vi "LM Numeric Gradient.vi"(6 "order":i32(ring)=1 items=["ORDER 1"=1, "ORDER 2"=2, "ORDER 4"=4], 7 "model function":T1, 8 "error in (no error)":errorcluster, 9 "X":dbl[](array[numeric]), 10 "f(X)":dbl[](array[numeric]), 11 "a":dbl[](array[numeric])) -> (0 "error out":errorcluster, 2 "number of function evaluations":i32, 3 "gradient":dbl[][](array[numeric]))   [LabVIEW 2010, in "NI_Gmath.lvlib"]
uses:
  NI_Gmath.lvlib
  LM model function.ctl
  LM model function reference.ctl
  LM_output select.ctl
  fpuIEEE64_finiteDiffConstants.ctl
panel:
  in  "stepsize (h)":dbl
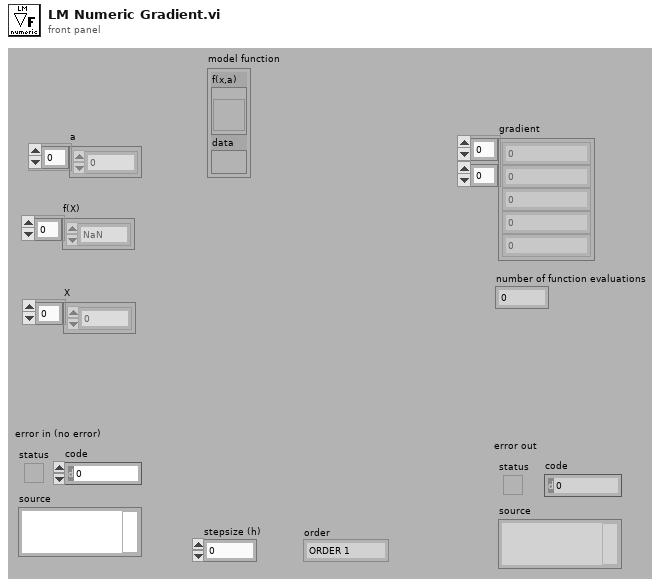
[diagram p1: front panel]
types:
  T1 = typedef "NI_Gmath.lvlib/LM model function.ctl" = cluster{"f(x,a)":T2, "data":variant}
  T2 = typedef "NI_Gmath.lvlib/LM model function reference.ctl" = refnum<vi>
  T3 = typedef "NI_Gmath.lvlib/LM_output select.ctl" = cluster{"model function":bool, "gradient":bool}
  T4 = typedef "NI_Gmath.lvlib/fpuIEEE64_finiteDiffConstants.ctl" = dbl
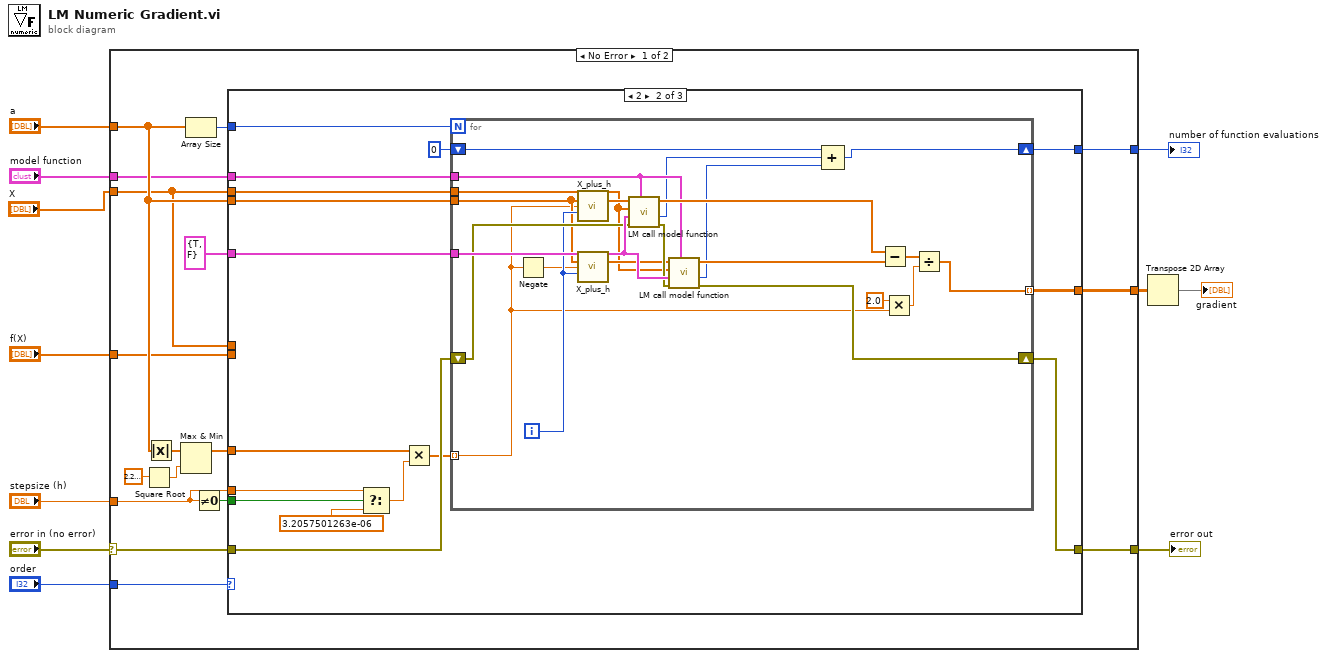
[diagram p0: block diagram]
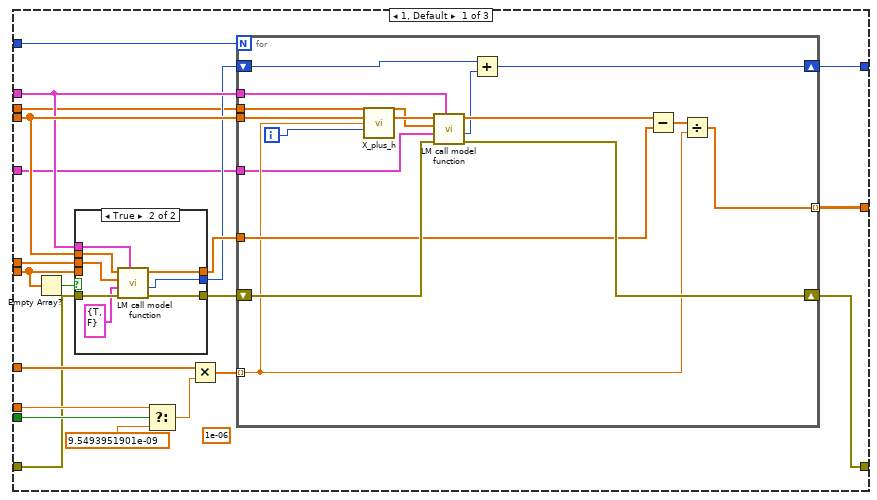
[diagram p2: hidden frame]
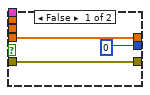
[diagram p3: hidden frame]
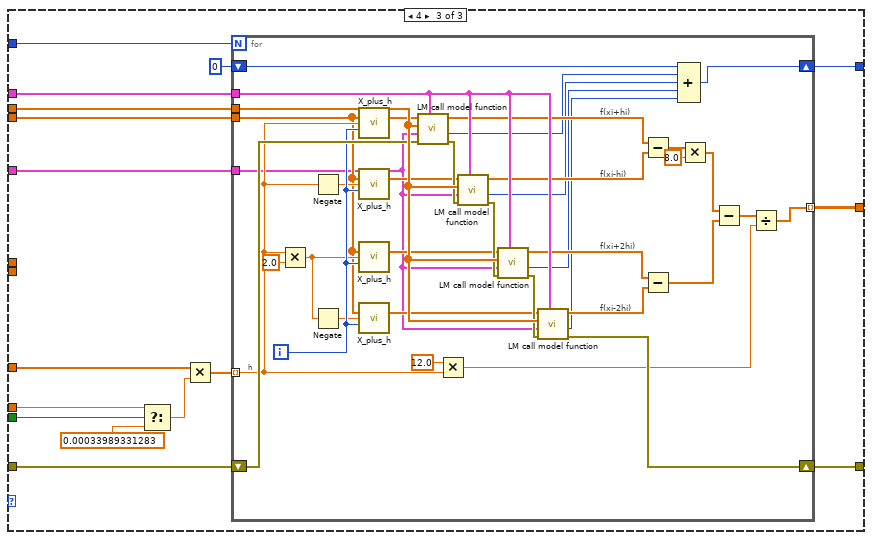
[diagram p4: hidden frame]
diagram:
  n1 = case shown="No Error" "error in (no error)" {
    selector: "error in (no error)" -> [w20 w168]
    tunnel: "a" -> [w28 _]
    tunnel: [w27 _] -> w10
    tunnel: "order" -> [w26 _]
    tunnel: "f(X)" -> [w24 _]
    tunnel: "stepsize (h)" -> [w23 _]
    tunnel: [w21 w168] -> w6
    tunnel: "model function" -> [w19 _]
    tunnel: [w18 _] -> w3
    tunnel: "X" -> [w17 _]
    frame No Error {
      n2 = Square Root(x=2.220446049250313e-16) -> (sqrt(x)=w14:dbl)
      n3 = Absolute Value(x=w28) -> (abs(x)=w13:dbl[])
      n4 = Max & Min(x=w13, y=w14) -> (max(x,y)=w12:dbl[])  [unwired: 1 out]
      n5 = Array Size(array=w28) -> (size(s)=w25:i32)
      n6 = Not Equal To 0?(x=w23) -> (x != 0?=w22:bool)
      n7 = case shown="2" w26 {
        tunnel: w28 -> [w45 w91 w130]
        tunnel: w20 -> [w38 w92 w121]
        tunnel: [w48 w90 w129] -> w27
        tunnel: w25 -> [w47 w89 w128]
        tunnel: w24 -> [w31 _ _]
        tunnel: w23 -> [w44 w86 w126]
        tunnel: w22 -> [w43 w87 w125]
        tunnel: w12 -> [w40 w85 w123]
        tunnel: [w49 w82 w120] -> w21
        tunnel: w19 -> [w37 w81 w119]
        tunnel: [w36 w79 w118] -> w18
        tunnel: w17 -> [w34 _ _]
        tunnel: w17 -> [w33 w78 w116]
        tunnel: T3 {"model function"=TRUE, "gradient"=FALSE} ("output control") -> [w30 w77 w115]
        frame 1, Default {
          (unwired) 1e-06
          w42 = T4 9.5493951901e-09 items=["H_FINITE_DIFF_1"=9.5493951901e-09, "H_FINITE_DIFF_2"=3.2057501263e-06, "H_FINITE_DIFF_4"=0.00033989331283, "H_FINITE_DIFF_K_1"=2.8120287999e-06, "H_FINITE_DIFF_K_2"=9.1341513557e-05, "H_FINITE_DIFF_K_3"=0.00045180790895, "H_FINITE_DIFF_K_4"=0.0014917421406] ("fpuIEEE64")
          n8 = Empty Array?(array=w31) -> (empty?=w32:bool)
          n9 = case shown="True" w32 {
            tunnel: [w52 w58] -> w46
            tunnel: w45 -> [_ w56]
            tunnel: w31 -> [w52 _]
            tunnel: w38 -> [w51 w60]
            tunnel: [w51 w59] -> w39
            tunnel: w37 -> [_ w57]
            tunnel: [0 ("number of function evaluations") w54] -> w35
            tunnel: w34 -> [_ w55]
            frame False {
            }
            frame True {
              n10 = call "LM call model function.vi"("model function"=w57, "error in (no error)"=w60, "output control"=T3 {"model function"=TRUE, "gradient"=FALSE}, "X"=w55, "a"=w56) -> ("error out"=w59:errorcluster, "number of function evaluations"=w54:i32, "f(X)"=w58:dbl[])  [unwired: 3 in, 1 out]
            }
          }
          n11 = Select(t=w44, s=w43, f=w42) -> (s? t:f=w41:T4)
          n12 = Multiply(x=w40, y=w41) -> (x*y=w29:T4[])
          n13 = for {
            N: w47 -> [_]
            tunnel: w45 -> [w70]
            tunnel: [w74] -> w48 mode=indexing
            tunnel: w46 -> [w72]
            tunnel: w29 -> [w69] mode=indexing
            shift-right: [w75] -> w49
            shift-left: w39 -> [w76]
            tunnel: w37 -> [w66]
            shift-right: [w64] -> w36
            shift-left: w35 -> [w65]
            tunnel: w33 -> [w63]
            tunnel: w30 -> [w61]
            i -> [w71]
            n14 = call "X_plus_h.vi"("X"=w70, "h"=w69, "i"=w71) -> ("Xi+h"=w68:dbl[])  [unwired: 12 in]
            n15 = call "LM call model function.vi"("model function"=w66, "error in (no error)"=w76, "output control"=w61, "X"=w63, "a"=w68) -> ("error out"=w75:errorcluster, "number of function evaluations"=w62:i32, "f(X)"=w67:dbl[])  [unwired: 3 in, 1 out]
            n16 = Add(x=w65, y=w62) -> (x+y=w64:i32)
            n17 = Subtract(x=w67, y=w72) -> (x-y=w73:dbl[])
            n18 = Divide(x=w73, y=w69) -> (x/y=w74:T4[])
          }
        }
        frame 2 {
          w88 = T4 3.2057501263e-06 items=["H_FINITE_DIFF_1"=9.5493951901e-09, "H_FINITE_DIFF_2"=3.2057501263e-06, "H_FINITE_DIFF_4"=0.00033989331283, "H_FINITE_DIFF_K_1"=2.8120287999e-06, "H_FINITE_DIFF_K_2"=9.1341513557e-05, "H_FINITE_DIFF_K_3"=0.00045180790895, "H_FINITE_DIFF_K_4"=0.0014917421406] ("fpuIEEE64")
          n19 = Select(t=w86, s=w87, f=w88) -> (s? t:f=w84:T4)
          n20 = Multiply(x=w85, y=w84) -> (x*y=w83:T4[])
          n21 = for {
            N: w89 -> [_]
            tunnel: w91 -> [w105]
            tunnel: [w107] -> w90 mode=indexing
            tunnel: w83 -> [w104] mode=indexing
            shift-right: [w112] -> w82
            shift-left: w92 -> [w111]
            tunnel: w81 -> [w100]
            shift-right: [w98] -> w79
            shift-left: 0 -> [w99]
            tunnel: w78 -> [w95]
            tunnel: w77 -> [w114]
            i -> [w110]
            n22 = Negate(x=w104) -> (-x=w103:T4)
            n23 = call "X_plus_h.vi"("X"=w105, "h"=w104, "i"=w110) -> ("Xi+h"=w96:dbl[])  [unwired: 12 in]
            n24 = call "X_plus_h.vi"("X"=w105, "h"=w103, "i"=w110) -> ("Xi+h"=w97:dbl[])  [unwired: 12 in]
            n25 = call "LM call model function.vi"("model function"=w100, "error in (no error)"=w111, "output control"=w114, "X"=w95, "a"=w96) -> ("error out"=w113:errorcluster, "number of function evaluations"=w94:i32, "f(X)"=w102:dbl[])  [unwired: 3 in, 1 out]
            n26 = call "LM call model function.vi"("model function"=w100, "error in (no error)"=w113, "output control"=w114, "X"=w95, "a"=w97) -> ("error out"=w112:errorcluster, "number of function evaluations"=w93:i32, "f(X)"=w101:dbl[])  [unwired: 3 in, 1 out]
            n27 = Compound Arithmetic op=ADD(w99, w94, w93) -> (w98:i32)
            n28 = Subtract(x=w102, y=w101) -> (x-y=w106:dbl[])
            n29 = Multiply(x=2.0, y=w104) -> (x*y=w108:T4)
            n30 = Divide(x=w106, y=w108) -> (x/y=w107:T4[])
          }
        }
        frame 4 {
          w127 = T4 0.00033989331283 items=["H_FINITE_DIFF_1"=9.5493951901e-09, "H_FINITE_DIFF_2"=3.2057501263e-06, "H_FINITE_DIFF_4"=0.00033989331283, "H_FINITE_DIFF_K_1"=2.8120287999e-06, "H_FINITE_DIFF_K_2"=9.1341513557e-05, "H_FINITE_DIFF_K_3"=0.00045180790895, "H_FINITE_DIFF_K_4"=0.0014917421406] ("fpuIEEE64")
          n31 = Select(t=w126, s=w125, f=w127) -> (s? t:f=w124:T4)
          n32 = Multiply(x=w123, y=w124) -> (x*y=w122:T4[])
          n33 = for {
            N: w128 -> [_]
            tunnel: w130 -> [w146]
            tunnel: [w152] -> w129 mode=indexing
            tunnel: w122 -> [w149] mode=indexing
            shift-right: [w164] -> w120
            shift-left: w121 -> [w165]
            tunnel: w119 -> [w166]
            shift-right: [w140] -> w118
            shift-left: 0 -> [w141]
            tunnel: w116 -> [w167]
            tunnel: w115 -> [w131]
            i -> [w160]
            # "h"
            # "f(xi-2hi)"
            # "f(xi+2hi)"
            # "f(xi-hi)"
            # "f(xi+hi)"
            n34 = Multiply(x=w149, y=2.0) -> (x*y=w147:T4)
            n35 = Negate(x=w149) -> (-x=w151:T4)
            n36 = Negate(x=w147) -> (-x=w148:T4)
            n37 = call "X_plus_h.vi"("X"=w146, "h"=w149, "i"=w160) -> ("Xi+h"=w139:dbl[])  [unwired: 12 in]
            n38 = call "X_plus_h.vi"("X"=w146, "h"=w151, "i"=w160) -> ("Xi+h"=w138:dbl[])  [unwired: 12 in]
            n39 = call "X_plus_h.vi"("X"=w146, "h"=w147, "i"=w160) -> ("Xi+h"=w137:dbl[])  [unwired: 12 in]
            n40 = call "X_plus_h.vi"("X"=w146, "h"=w148, "i"=w160) -> ("Xi+h"=w136:dbl[])  [unwired: 12 in]
            n41 = call "LM call model function.vi"("model function"=w166, "error in (no error)"=w165, "output control"=w131, "X"=w167, "a"=w139) -> ("error out"=w161:errorcluster, "number of function evaluations"=w135:i32, "f(X)"=w145:dbl[])  [unwired: 3 in, 1 out]
            n42 = Multiply(x=12.0, y=w149) -> (x*y=w154:T4)
            n43 = call "LM call model function.vi"("model function"=w166, "error in (no error)"=w161, "output control"=w131, "X"=w167, "a"=w138) -> ("error out"=w162:errorcluster, "number of function evaluations"=w134:i32, "f(X)"=w144:dbl[])  [unwired: 3 in, 1 out]
            n44 = call "LM call model function.vi"("model function"=w166, "error in (no error)"=w162, "output control"=w131, "X"=w167, "a"=w137) -> ("error out"=w163:errorcluster, "number of function evaluations"=w133:i32, "f(X)"=w143:dbl[])  [unwired: 3 in, 1 out]
            n45 = call "LM call model function.vi"("model function"=w166, "error in (no error)"=w163, "output control"=w131, "X"=w167, "a"=w136) -> ("error out"=w164:errorcluster, "number of function evaluations"=w132:i32, "f(X)"=w142:dbl[])  [unwired: 3 in, 1 out]
            n46 = Subtract(x=w145, y=w144) -> (x-y=w158:dbl[])
            n47 = Subtract(x=w143, y=w142) -> (x-y=w155:dbl[])
            n48 = Compound Arithmetic op=ADD(w141, w135, w134, w133, w132) -> (w140:i32)
            n49 = Multiply(x=w158, y=8.0) -> (x*y=w156:dbl[])
            n50 = Subtract(x=w156, y=w155) -> (x-y=w153:dbl[])
            n51 = Divide(x=w153, y=w154) -> (x/y=w152:T4[])
          }
        }
      }
    }
    frame Error {
    }
  }
  "error out" <- w6
  "number of function evaluations" <- w3
  n52 = Transpose 2D Array(2D array=w10) -> (transposed array=→"gradient":T4[][])
